vi "Mouse Read.vi"(3 "Read Address":u8 format="%x", 4 "Timeout (ms)":i32=100, 5 "FPGA VI Reference In":refnum<k20>) -> (0 "Timed out?":bool, 1 "Read Data out":u8, 2 "FPGA VI Reference Out":refnum<k20>)   [LabVIEW 2012]
uses:
  <vilib>/Utility/error.llb/Error Cluster From Error Code.vi
  <vilib>/rvi/errors/niLvFpgaAdjustHostInterfaceError.vi
  <vilib>/rvi/interface/nirviReadWriteControl/nirviReadWriteControl.xnode
  NiFpgaLv.dll
  <vilib>/rvi/interface/Simulation/niFpgaSimulationCallBeginRW.vi
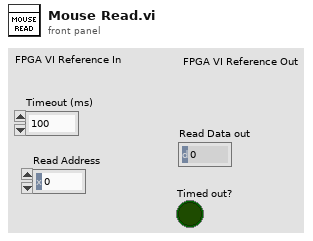
[diagram p1: front panel]
types:
  T1 = enum16{"idle", "set idle", "begin", "write", "read", "power down", "reset"}
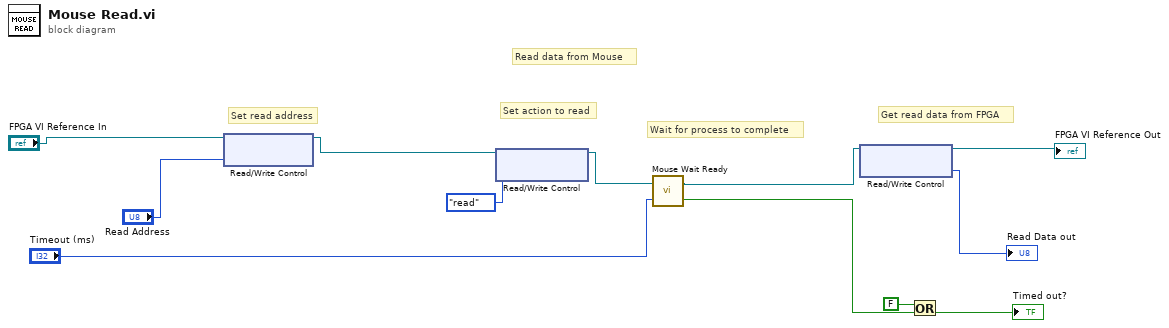
[diagram p0: block diagram]
diagram:
  # "Get read data from FPGA"
  # "Wait for process to complete"
  # "Set read address"
  # "Set action to read"
  # "Read data from Mouse"
  n1 = xnode "Read/Write Control"("FPGA VI Reference In"="FPGA VI Reference In", "Read Address"="Read Address") -> ("FPGA VI Reference Out"=w2:refnum<k20>)  [unwired: 1 in, 1 out]
  n2 = xnode "Read/Write Control"("FPGA VI Reference In"=w2, "Mouse Action"=T1."read") -> ("FPGA VI Reference Out"=w1:refnum<k20>)  [unwired: 1 in, 1 out]
  n3 = call "Mouse Wait Ready.vi"("Timeout (ms)"="Timeout (ms)", "Refnum in"=w1) -> ("Timeout"=w7:bool, "Refnum out"=w8:refnum<k20>)
  n4 = xnode "Read/Write Control"("FPGA VI Reference In"=w8) -> ("FPGA VI Reference Out"=→"FPGA VI Reference Out":refnum<k20>, "Read Data out"=→"Read Data out":u8)  [unwired: 1 in, 1 out]
  n5 = Or(x=FALSE, y=w7) -> (x .or. y?=→"Timed out?":bool)
